vi "CANOpen_Log Init Cluster.vi"(8 "error in":errorcluster, 9 "Write?":bool=TRUE, 10 "datalog path":path=path "c:/init cluster.dat", 11 "cluster 2":T25={"Device Error"={"status"=FALSE, "code"=0, "source"=""}, "Error Handling Cluster"={"Error Process Q"=refnum, "Process Qs"=[]}, "VI Ref In"=[], "CD Settings"={"Driver Settings"={"CANOpen Bus Settings"={"CANOpen Interface Name"=0, "Baud Rate"=0, "Termination"=FALSE, "Sync Period (ms)"=10, "Enable 9881"=FALSE, "RIO Device"=0, "Enable SYNC"=FALSE, "Scan & Print"=FALSE}, "Nodes"=[], "Node Ids"=[]}, "Data References"={"Hardware Input"={"FIFO"=refnum, "Channel Pairs"={"Chan Refs"=[], "Prev. Values"=[]}}, "Hardware Output"={"FIFO"=refnum, "Channel Pairs"={"Block Refs"=[], "Prev. Values"=[]}}}, "Bus Commands"={"Hardware Output"={"FIFO"=refnum, "Channel Pairs"={"Chan Refs"=[], "Prev. Values"=[]}}, "Hardware Input"={"FIFO"=refnum}}, "SDO Asynch"={"List SDO"={"FIFO Req"=refnum, "Req Chan."={"Chan Refs"=[], "NodeIndex"=[]}, "FIFO Resp"=refnum, "Resp Chan."={"Chan Refs"=[]}, "Node IDs"=[], "FIFO array"=[]}, "HW Dyn Write"={"FIFO Req"=refnum, "FIFO Resp"=refnum, "Req Chan."={"Chan Refs"=[], "Node IDs"=[]}, "Resp Chan."={"Chan Refs"=[]}}, "HW Dyn Read"={"FIFO Req"=refnum, "FIFO Resp"=refnum, "Req Chan."={"Chan Refs"=[], "Node IDs"=[]}, "Resp Chan."={"Chan Refs"=[]}}}, "Status NMT"={"Hardware Output"={"FIFO"=refnum, "Channel Pairs"={"Chan Refs"=[], "Prev. Values"=[], "Node index"=[]}}, "Hardware Input"={"FIFO"=refnum, "Channel Pairs"={"Chan Refs"=[], "Prev. Values"=[], "Node index"=[]}}}}, "FPGA Session"=0} {"CD Settings"."Status NMT"."Hardware Output"."Channel Pairs"."Chan Refs"."Data Reference" format="%.0x"; "CD Settings"."Status NMT"."Hardware Input"."Channel Pairs"."Chan Refs" format="%.0x"; "CD Settings"."SDO Asynch"."HW Dyn Read"."Resp Chan."."Chan Refs" format="%.0x"; "CD Settings"."SDO Asynch"."HW Dyn Read"."Req Chan."."Chan Refs" format="%.0x"; "CD Settings"."SDO Asynch"."HW Dyn Write"."Resp Chan."."Chan Refs" format="%.0x"; "CD Settings"."SDO Asynch"."HW Dyn Write"."Req Chan."."Chan Refs" format="%.0x"; "CD Settings"."SDO Asynch"."List SDO"."Resp Chan."."Chan Refs" format="%.0x"; "CD Settings"."SDO Asynch"."List SDO"."Req Chan."."Chan Refs" format="%.0x"; "CD Settings"."Bus Commands"."Hardware Output"."Channel Pairs"."Chan Refs" format="%.0x"; "CD Settings"."Data References"."Hardware Input"."Channel Pairs"."Chan Refs" format="%.0x"; "CD Settings"."Data References"."Hardware Output"."Channel Pairs"."Block Refs"."Data Reference" format="%.0x"; "CD Settings"."Driver Settings"."CANOpen Bus Settings"."Baud Rate" items=["1 Mbit/s"=0, "800 kbit/s"=1, "500 kbit/s"=2, "250 kbit/s"=3, "125 kbit/s"=4, "50 kbit/s"=6, "20 kbit/s"=7, "10 kbit/s"=8]; "CD Settings"."Driver Settings"."CANOpen Bus Settings"."CANOpen Interface Name" items=["CANopen01", "CANopen02", "CANopen03", "CANopen04", "CANopen05", "CANopen06", "CANopen07", "CANopen08", "CANopen09", "CANopen10", "CANopen11", "CANopen12", "CANopen13", "CANopen14", "CANopen15", "CANopen16", "CANopen17", "CANopen18", "CANopen19", "CANopen20", "CANopen21", "CANopen22", "CANopen23", "CANopen24", "CANopen25", "CANopen26", "CANopen27", "CANopen28", "CANopen29", "CANopen30", "CANopen31", "CANopen32"]; "CD Settings"."Driver Settings"."Nodes"."NMT"."Node init static SDO state" items=["start remote node"=1, "enter pre-operational"=128]; "CD Settings"."Driver Settings"."Nodes"."NMT"."Node run state" items=["start remote node"=1, "stop remote node"=2, "enter pre-operational"=128, "reset node"=129, "reset communication"=130]; "CD Settings"."Driver Settings"."Nodes"."Dynamic SDOs"."Sub-Index (0)" format="%.0x"; "CD Settings"."Driver Settings"."Nodes"."Dynamic SDOs"."Object Index" format="%.0x"; "CD Settings"."Driver Settings"."Nodes"."Dynamic SDOs"."Block Data" format="%.0x"; "CD Settings"."Driver Settings"."Nodes"."RPDOs"."PDO Channel" items=["PDO 1", "PDO 2", "PDO 3", "PDO 4"]; "CD Settings"."Driver Settings"."Nodes"."TPDOs"."PDO Channel" items=["PDO 1", "PDO 2", "PDO 3", "PDO 4"]; "CD Settings"."Driver Settings"."Nodes"."SDOs"."Sub-Index (0)" format="%.0x"; "CD Settings"."Driver Settings"."Nodes"."SDOs"."Object Index" format="%.0x"; "CD Settings"."Driver Settings"."Nodes"."SDOs"."Block Data" format="%.0x"}) -> (0 "error out":errorcluster, 3 "cluster 2":T25={"Device Error"={"status"=FALSE, "code"=0, "source"=""}, "Error Handling Cluster"={"Error Process Q"=refnum, "Process Qs"=[]}, "VI Ref In"=[], "CD Settings"={"Driver Settings"={"CANOpen Bus Settings"={"CANOpen Interface Name"=0, "Baud Rate"=0, "Termination"=FALSE, "Sync Period (ms)"=10, "Enable 9881"=FALSE, "RIO Device"=0, "Enable SYNC"=FALSE, "Scan & Print"=FALSE}, "Nodes"=[], "Node Ids"=[]}, "Data References"={"Hardware Input"={"FIFO"=refnum, "Channel Pairs"={"Chan Refs"=[], "Prev. Values"=[]}}, "Hardware Output"={"FIFO"=refnum, "Channel Pairs"={"Block Refs"=[], "Prev. Values"=[]}}}, "Bus Commands"={"Hardware Output"={"FIFO"=refnum, "Channel Pairs"={"Chan Refs"=[], "Prev. Values"=[]}}, "Hardware Input"={"FIFO"=refnum}}, "SDO Asynch"={"List SDO"={"FIFO Req"=refnum, "Req Chan."={"Chan Refs"=[], "NodeIndex"=[]}, "FIFO Resp"=refnum, "Resp Chan."={"Chan Refs"=[]}, "Node IDs"=[], "FIFO array"=[]}, "HW Dyn Write"={"FIFO Req"=refnum, "FIFO Resp"=refnum, "Req Chan."={"Chan Refs"=[], "Node IDs"=[]}, "Resp Chan."={"Chan Refs"=[]}}, "HW Dyn Read"={"FIFO Req"=refnum, "FIFO Resp"=refnum, "Req Chan."={"Chan Refs"=[], "Node IDs"=[]}, "Resp Chan."={"Chan Refs"=[]}}}, "Status NMT"={"Hardware Output"={"FIFO"=refnum, "Channel Pairs"={"Chan Refs"=[], "Prev. Values"=[], "Node index"=[]}}, "Hardware Input"={"FIFO"=refnum, "Channel Pairs"={"Chan Refs"=[], "Prev. Values"=[], "Node index"=[]}}}}, "FPGA Session"=0} {"CD Settings"."Status NMT"."Hardware Output"."Channel Pairs"."Chan Refs"."Data Reference" format="%.0x"; "CD Settings"."Status NMT"."Hardware Input"."Channel Pairs"."Chan Refs" format="%.0x"; "CD Settings"."SDO Asynch"."HW Dyn Read"."Resp Chan."."Chan Refs" format="%.0x"; "CD Settings"."SDO Asynch"."HW Dyn Read"."Req Chan."."Chan Refs" format="%.0x"; "CD Settings"."SDO Asynch"."HW Dyn Write"."Resp Chan."."Chan Refs" format="%.0x"; "CD Settings"."SDO Asynch"."HW Dyn Write"."Req Chan."."Chan Refs" format="%.0x"; "CD Settings"."SDO Asynch"."List SDO"."Resp Chan."."Chan Refs" format="%.0x"; "CD Settings"."SDO Asynch"."List SDO"."Req Chan."."Chan Refs" format="%.0x"; "CD Settings"."Bus Commands"."Hardware Output"."Channel Pairs"."Chan Refs" format="%.0x"; "CD Settings"."Data References"."Hardware Input"."Channel Pairs"."Chan Refs" format="%.0x"; "CD Settings"."Data References"."Hardware Output"."Channel Pairs"."Block Refs"."Data Reference" format="%.0x"; "CD Settings"."Driver Settings"."CANOpen Bus Settings"."Baud Rate" items=["1 Mbit/s"=0, "800 kbit/s"=1, "500 kbit/s"=2, "250 kbit/s"=3, "125 kbit/s"=4, "50 kbit/s"=6, "20 kbit/s"=7, "10 kbit/s"=8]; "CD Settings"."Driver Settings"."CANOpen Bus Settings"."CANOpen Interface Name" items=["CANopen01", "CANopen02", "CANopen03", "CANopen04", "CANopen05", "CANopen06", "CANopen07", "CANopen08", "CANopen09", "CANopen10", "CANopen11", "CANopen12", "CANopen13", "CANopen14", "CANopen15", "CANopen16", "CANopen17", "CANopen18", "CANopen19", "CANopen20", "CANopen21", "CANopen22", "CANopen23", "CANopen24", "CANopen25", "CANopen26", "CANopen27", "CANopen28", "CANopen29", "CANopen30", "CANopen31", "CANopen32"]; "CD Settings"."Driver Settings"."Nodes"."NMT"."Node init static SDO state" items=["start remote node"=1, "enter pre-operational"=128]; "CD Settings"."Driver Settings"."Nodes"."NMT"."Node run state" items=["start remote node"=1, "stop remote node"=2, "enter pre-operational"=128, "reset node"=129, "reset communication"=130]; "CD Settings"."Driver Settings"."Nodes"."Dynamic SDOs"."Sub-Index (0)" format="%.0x"; "CD Settings"."Driver Settings"."Nodes"."Dynamic SDOs"."Object Index" format="%.0x"; "CD Settings"."Driver Settings"."Nodes"."Dynamic SDOs"."Block Data" format="%.0x"; "CD Settings"."Driver Settings"."Nodes"."RPDOs"."PDO Channel" items=["PDO 1", "PDO 2", "PDO 3", "PDO 4"]; "CD Settings"."Driver Settings"."Nodes"."TPDOs"."PDO Channel" items=["PDO 1", "PDO 2", "PDO 3", "PDO 4"]; "CD Settings"."Driver Settings"."Nodes"."SDOs"."Sub-Index (0)" format="%.0x"; "CD Settings"."Driver Settings"."Nodes"."SDOs"."Object Index" format="%.0x"; "CD Settings"."Driver Settings"."Nodes"."SDOs"."Block Data" format="%.0x"})   [LabVIEW 2021, in "CANOpen Addon Engine.lvlib"]
uses:
  CANOpen Addon Engine.lvlib
  Error Handling API/_Controls/VS Errors_Error Handling Cluster.ctl
  CANOpen_Settings.ctl
  CANOpen_Node Settings.ctl
  Shared/CANOpen_Bus Settings.ctl
  Shared/CANOpen Interface Name.ctl
  <vilib>/CANopenLib/CANOPEN.llb/CANopen BaudRate.ctl
  CANOpen_Node Message Settings.ctl
  Shared/CANOpen_PDO Settings.ctl
  Shared/CANOpen_PDO Parameter Settings.ctl
  Shared/CANOpen_PDO Data Type.ctl
  Shared/CANopen Byte Order.ctl
  Shared/CANOpen_SDO Settings.ctl
  CANOpen_NMT Settings.ctl
  Shared/CanOpen_NMT_Config.ctl
  Shared/CanOpen_NMT_Static detect.ctl
  Async VIs/CANOpen_Main/SubVIs/CanOpen_Main Node Ids.ctl
  CANOpen_VS Data Refs.ctl
  <vilib>/NI VeriStand/Custom Device API/Data Reference.ctl
  <vilib>/NI VeriStand/Custom Device API/Block Data Reference.ctl
  CANOpen_VS Bidirectional Data Refs.ctl
  CANOpen_VS SDOs Data Refs.ctl
  Async VIs/CANOpen_Main/SubVIs/CanOpen_SDO Dynamic queue.ctl
  Shared/CANOpen_SDO queue W data.ctl
  Shared/CANOpen_SDO queue mode.ctl
  Shared/CANOpen_PDO Data Type in queue.ctl
  CANOpen_VS Status Management Data Refs.ctl
  Async VIs/CANOpen_Main/SubVIs/CanOpen_NMT_HWOut_ChannelPairs.ctl
  Async VIs/CANOpen_Main/SubVIs/CanOpen_NMT_HWIn_ChannelPairs.ctl
  <vilib>/NI VeriStand/Custom Device API/Custom Device API.lvlib
  Shared/CANOpen Addon Shared.lvlib
panel:
  # "LSB"
  # "MSB"
  # "LSB"
  # "MSB"
  # "LSB"
  # "MSB"
  # "LSB"
  # "MSB"
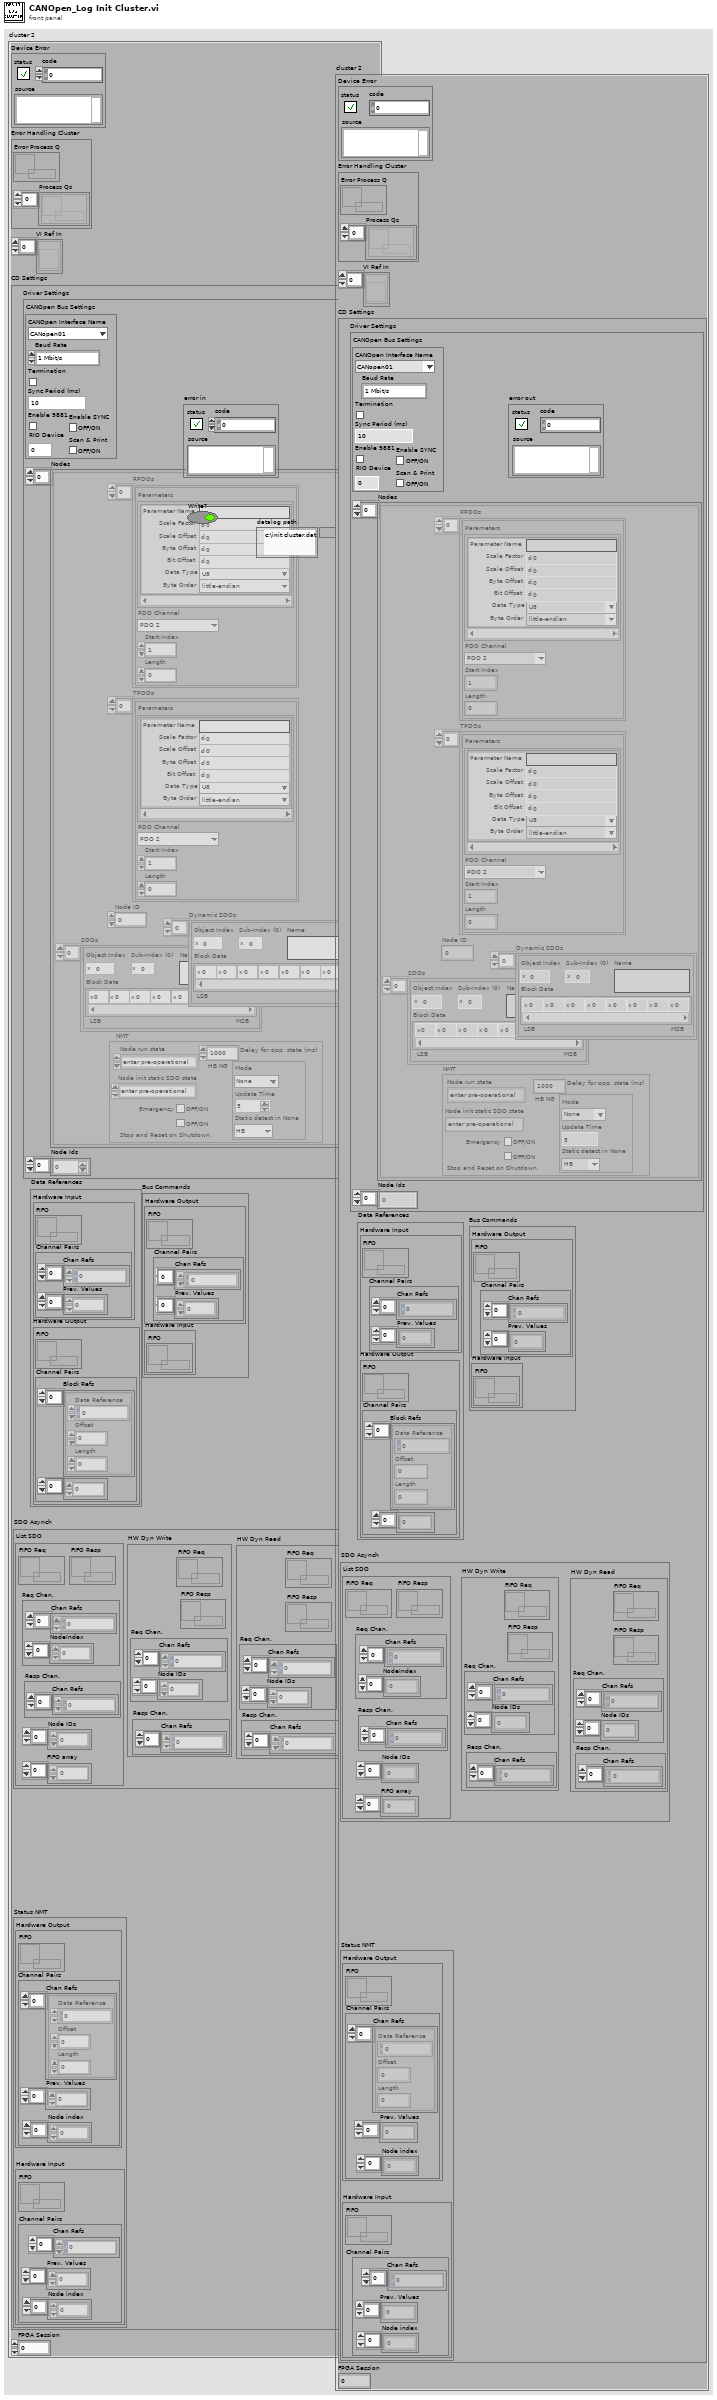
[diagram p1: front panel]
types:
  T1 = typedef "CANOpen Addon Engine.lvlib/VS Errors_Error Handling Cluster.ctl" = cluster{"Error Process Q":refnum<queue>, "Process Qs":refnum<queue>[]}
  T2 = typedef "CANOpen Addon Engine.lvlib/CANOpen_Settings.ctl" = cluster{"Driver Settings":T3, "Data References":T17, "Bus Commands":T20, "SDO Asynch":T21, "Status NMT":T22}
  T3 = typedef "CANOpen Addon Engine.lvlib/CANOpen_Node Settings.ctl" = cluster{"CANOpen Bus Settings":T4, "Nodes":T7[], "Node Ids":T16}
  T4 = typedef "CANOpen Addon Shared.lvlib/CANOpen_Bus Settings.ctl" = cluster{"CANOpen Interface Name":T5, "Baud Rate":T6, "Termination":bool, "Sync Period (ms)":i64, "Enable 9881":bool, "RIO Device":u16, "Enable SYNC":bool, "Scan & Print":bool}
  T5 = typedef "CANOpen Addon Shared.lvlib/CANOpen Interface Name.ctl" = u32
  T6 = typedef "CANopen BaudRate.ctl" = u32
  T7 = typedef "CANOpen Addon Engine.lvlib/CANOpen_Node Message Settings.ctl" = cluster{"RPDOs":T8[], "TPDOs":T8[], "Node ID":u8, "SDOs":T12[], "Dynamic SDOs":T12[], "NMT":T13}
  T8 = typedef "CANOpen Addon Shared.lvlib/CANOpen_PDO Settings.ctl" = cluster{"Parameters":T9[], "PDO Channel":u8, "Start Index":u32, "Length":u32}
  T9 = typedef "CANOpen Addon Shared.lvlib/CANOpen_PDO Parameter Settings.ctl" = cluster{"Parameter Name":string, "Scale Factor":dbl, "Scale Offset":dbl, "Byte Offset":u8, "Bit Offset":u8, "Data Type":T10, "Byte Order":T11}
  T10 = typedef "CANOpen Addon Shared.lvlib/CANOpen_PDO Data Type.ctl" = enum16{"U8", "U16", "U32", "I8", "I16", "I32", "Single", "Double", "Boolean"}
  T11 = typedef "CANOpen Addon Shared.lvlib/CANopen Byte Order.ctl" = enum16{"big-endian network order", "little-endian"}
  T12 = typedef "CANOpen Addon Shared.lvlib/CANOpen_SDO Settings.ctl" = cluster{"Object Index":u16, "Sub-Index (0)":u8, "Block Data":u8[], "Name":string}
  T13 = typedef "CANOpen Addon Engine.lvlib/CANOpen_NMT Settings.ctl" = cluster{"Node run state":u16, "Emergency":bool, "HB NG":T14, "Delay for opp. state (ms)":dbl, "Node init static SDO state":u16, "Stop and Reset on Shutdown":bool}
  T14 = typedef "CANOpen Addon Shared.lvlib/CanOpen_NMT_Config.ctl" = cluster{"Mode":T15, "Update Time":u16, "Static detect in None":T15}
  T15 = typedef "CANOpen Addon Shared.lvlib/CanOpen_NMT_Static detect.ctl" = enum16{"None", "HB", "NG"}
  T16 = typedef "CANOpen Addon Engine.lvlib/CanOpen_Main Node Ids.ctl" = u8[]
  T17 = typedef "CANOpen Addon Engine.lvlib/CANOpen_VS Data Refs.ctl" = cluster{"Hardware Input":cluster{"FIFO":refnum<k33>, "Channel Pairs":cluster{"Chan Refs":T18[], "Prev. Values":dbl[]}}, "Hardware Output":cluster{"FIFO":refnum<k33>, "Channel Pairs":cluster{"Block Refs":T19[], "Prev. Values":dbl[]}}}
  T18 = typedef "Custom Device API.lvlib/Data Reference.ctl" = i32
  T19 = typedef "Custom Device API.lvlib/Block Data Reference.ctl" = cluster{"Data Reference":T18, "Offset":u64, "Length":u64}
  T20 = typedef "CANOpen Addon Engine.lvlib/CANOpen_VS Bidirectional Data Refs.ctl" = cluster{"Hardware Output":cluster{"FIFO":refnum<k33>, "Channel Pairs":cluster{"Chan Refs":T18[], "Prev. Values":dbl[]}}, "Hardware Input":cluster{"FIFO":refnum<k33>}}
  T21 = typedef "CANOpen Addon Engine.lvlib/CANOpen_VS SDOs Data Refs.ctl" = cluster{"List SDO":cluster{"FIFO Req":refnum<k33>, "Req Chan.":cluster{"Chan Refs":T18[], "NodeIndex":dbl[]}, "FIFO Resp":refnum<k33>, "Resp Chan.":cluster{"Chan Refs":T18[]}, "Node IDs":u8[], "FIFO array":dbl[]}, "HW Dyn Write":cluster{"FIFO Req":refnum<k33>, "FIFO Resp":refnum<k33>, "Req Chan.":cluster{"Chan Refs":T18[], "Node IDs":u8[]}, "Resp Chan.":cluster{"Chan Refs":T18[]}}, "HW Dyn Read":cluster{"FIFO Req":refnum<k33>, "FIFO Resp":refnum<k33>, "Req Chan.":cluster{"Chan Refs":T18[], "Node IDs":u8[]}, "Resp Chan.":cluster{"Chan Refs":T18[]}}}
  T22 = typedef "CANOpen Addon Engine.lvlib/CANOpen_VS Status Management Data Refs.ctl" = cluster{"Hardware Output":cluster{"FIFO":refnum<k33>, "Channel Pairs":T23}, "Hardware Input":cluster{"FIFO":refnum<k33>, "Channel Pairs":T24}}
  T23 = typedef "CANOpen Addon Engine.lvlib/CanOpen_NMT_HWOut_ChannelPairs.ctl" = cluster{"Chan Refs":T19[], "Prev. Values":dbl[], "Node index":dbl[]}
  T24 = typedef "CANOpen Addon Engine.lvlib/CanOpen_NMT_HWIn_ChannelPairs.ctl" = cluster{"Chan Refs":T18[], "Prev. Values":dbl[], "Node index":dbl[]}
  T25 = cluster{"Device Error":errorcluster, "Error Handling Cluster":T1, "VI Ref In":refnum<vi>[], "CD Settings":T2, "FPGA Session":u32}
  T26 = enum16{"open", "replace", "create", "open or create", "replace or create", "replace or create with confirmation"}
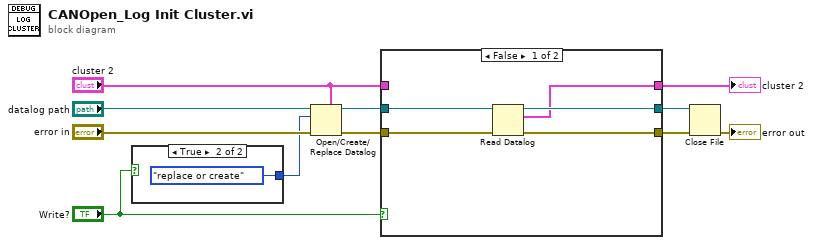
[diagram p0: block diagram]
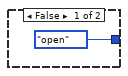
[diagram p2: hidden frame]
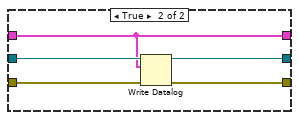
[diagram p3: hidden frame]
diagram:
  n1 = case shown="True" "Write?" {
    tunnel: [T26."open" ("operation (0:open)") T26."replace or create" ("operation (0:open)")] -> w4
    frame False {
    }
    frame True {
    }
  }
  n2 = Open/Create/Replace Datalog(5:"cluster 2", 8:"error in", 10:w4, 11:"datalog path") -> (0:w10:errorcluster, 3:w9:refnum<k1>)  [unwired: 2 in, 1 out]
  n3 = case shown="False" "Write?" {
    tunnel: [w15 w23] -> w11
    tunnel: w10 -> [w18 w22]
    tunnel: w9 -> [w17 w21]
    tunnel: [w16 w20] -> w8
    tunnel: "cluster 2" -> [_ w19]
    tunnel: [w14 w19] -> w3
    frame False {
      n4 = Read Datalog(4:w18, 7:w17) -> (0:w15:errorcluster, 2:w14:T25, 3:w16:refnum<k1>)  [unwired: 1 in]
    }
    frame True {
      n5 = Write Datalog(4:w22, 6:w19, 7:w21) -> (0:w23:errorcluster, 3:w20:refnum<k1>)
    }
  }
  "cluster 2" <- w3
  n6 = Close File(refnum=w8, error in=w11) -> (error out=→"error out":errorcluster)  [unwired: 1 out]
